vi "MGI Find Closest Line Segment.vi"(9 "Y":dbl, 10 "X":dbl, 11 "Graph Data":cluster{"X":dbl[], "Y":dbl[]}) -> (1 "Distance":dbl, 3 "Index of first point in line":i32)   [LabVIEW 2016]
doc: "Finds the line segment closest to the given x and y coordinates. The Graph Data is intepreted as a sequence of points which are connected by line segments. The points in the graph are assumed to be connected in the order provided. The output index is the index of the first point in the data that is an endpoint of the closest line segment.\n\nAuthored by Thomas E. Henage\nsupport@mooregoodideas.com\nwww.mooregoodideas.com\n\nCopyright (c) 2010, Moore Good Ideas, Inc.\n\nAll rights reserved.\n\nRedistribution and use in source and binary forms, with or without modification, are permitted provided that the following conditions are met:\n\n * Redistributions of source code must retain the above copyright notice, this list of conditions and the following disclaimer.\n * Redistributions in binary form must reproduce the above copyright notice, this list of conditions and the following disclaimer in the documentation and/or other materials provided with the distribution.\n * Neither the name of Moore Good Ideas, Inc. nor the names of its contributors may be used to endorse or promote products derived from this software without specific prior written permission.\n\nTHIS SOFTWARE IS PROVIDED BY THE COPYRIGHT HOLDERS AND CONTRIBUTORS \"AS IS\" AND ANY EXPRESS OR IMPLIED WARRANTIES, INCLUDING, BUT NOT LIMITED TO, THE IMPLIED WARRANTIES OF MERCHANTABILITY AND FITNESS FOR A PARTICULAR PURPOSE ARE DISCLAIMED. IN NO EVENT SHALL THE COPYRIGHT OWNER OR CONTRIBUTORS BE LIABLE FOR ANY DIRECT, INDIRECT, INCIDENTAL, SPECIAL, EXEMPLARY, OR CONSEQUENTIAL DAMAGES (INCLUDING, BUT NOT LIMITED TO, PROCUREMENT OF SUBSTITUTE GOODS OR SERVICES; LOSS OF USE, DATA, OR PROFITS; OR BUSINESS INTERRUPTION) HOWEVER CAUSED AND ON ANY THEORY OF LIABILITY, WHETHER IN CONTRACT, STRICT LIABILITY, OR TORT (INCLUDING NEGLIGENCE OR OTHERWISE) ARISING IN ANY WAY OUT OF THE USE OF THIS SOFTWARE, EVEN IF ADVISED OF THE POSSIBILITY OF SUCH DAMAGE."
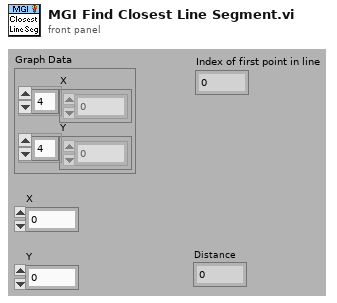
[diagram p1: front panel]
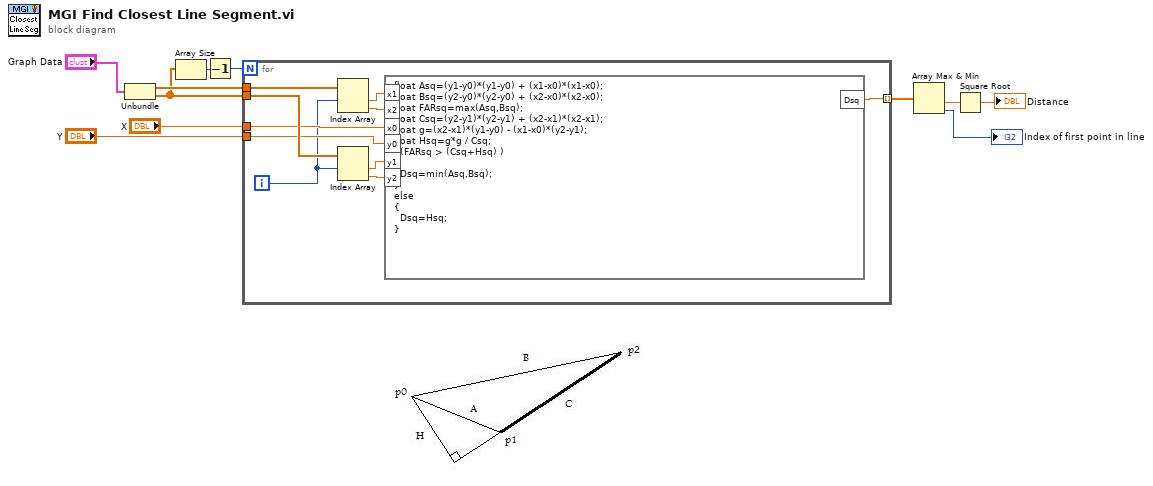
[diagram p0: block diagram]
diagram:
  n1 = Unbundle("Graph Data") -> ("X"=w7:dbl[], "Y"=w5:dbl[])
  n2 = Array Size(array=w5) -> (size(s)=w4:i32)
  n3 = Decrement(x=w4) -> (x-1=w3:i32)
  n4 = for {
    N: w3 -> [_]
    tunnel: w7 -> [w21]
    tunnel: w5 -> [w20]
    tunnel: "X" -> [w15]
    tunnel: "Y" -> [w14]
    tunnel: [w13] -> w10 mode=indexing
    i -> [w12]
    n5 = Index Array(array=w21, index #1=w12) -> (element #1=w19:dbl, element #2=w18:dbl)  [unwired: 1 in]
    n6 = Index Array(array=w20, index #1=w12) -> (element #1=w17:dbl, element #2=w16:dbl)  [unwired: 1 in]
    n7 = formula code="float Asq=(y1-y0)*(y1-y0) + (x1-x0)*(x1-x0);\nfloat Bsq=(y2-y0)*(y2-y0) + (x2-x0)*(x2-x0);\nfloat FARsq=max(Asq,Bsq);\nfloat Csq=(y2-y1)*(y2-y1) + (x2-x1)*(x2-x1);\nfloat g=(x2-x1)*(y1-y0) - (x1-x0)*(y2-y1);\nfloat Hsq=g*g / Csq;\nif(FARsq > (Csq+Hsq) )\n{\n  Dsq=min(Asq,Bsq);\n}\nelse\n{\n  Dsq=Hsq;\n}"("x1"=w19, "x2"=w18, "y1"=w17, "y2"=w16, "x0"=w15, "y0"=w14) -> ("Dsq"=w13:dbl)
  }
  n8 = Array Max & Min(array=w10) -> (min value=w2:dbl, min index (indices)=→"Index of first point in line":i32)  [unwired: 2 out]
  n9 = Square Root(x=w2) -> (sqrt(x)=→"Distance":dbl)
